vi "Login-Panel.vi"() -> ()   [LabVIEW 2021]
uses:
  <vilib>/lvdsc/security/NI Security Programmatic Login (Name).vi
  Global-Var-Simulator.vi
  <vilib>/lvdsc/NI_DSC.lvlib
panel:
  in  "goto_control_panel_btn":bool
  in  "logout_button":bool
  out "active_user_L":string
  in  "goto_service_panel_btn":bool
  in  "service_login_btn":bool
  in  "goto_wash_panel_btn":bool
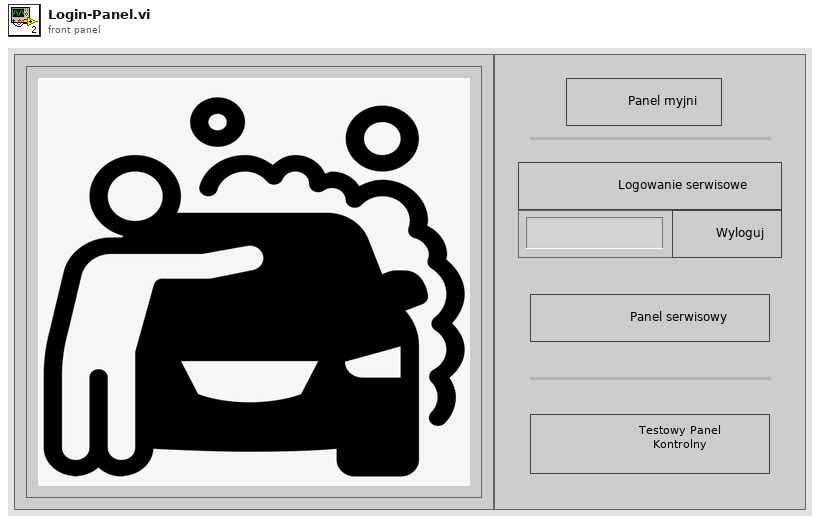
[diagram p1: front panel]
types:
  T1 = enum32{"Invalid", "Standard", "Closed", "Hidden", "Minimized", "Maximized"}
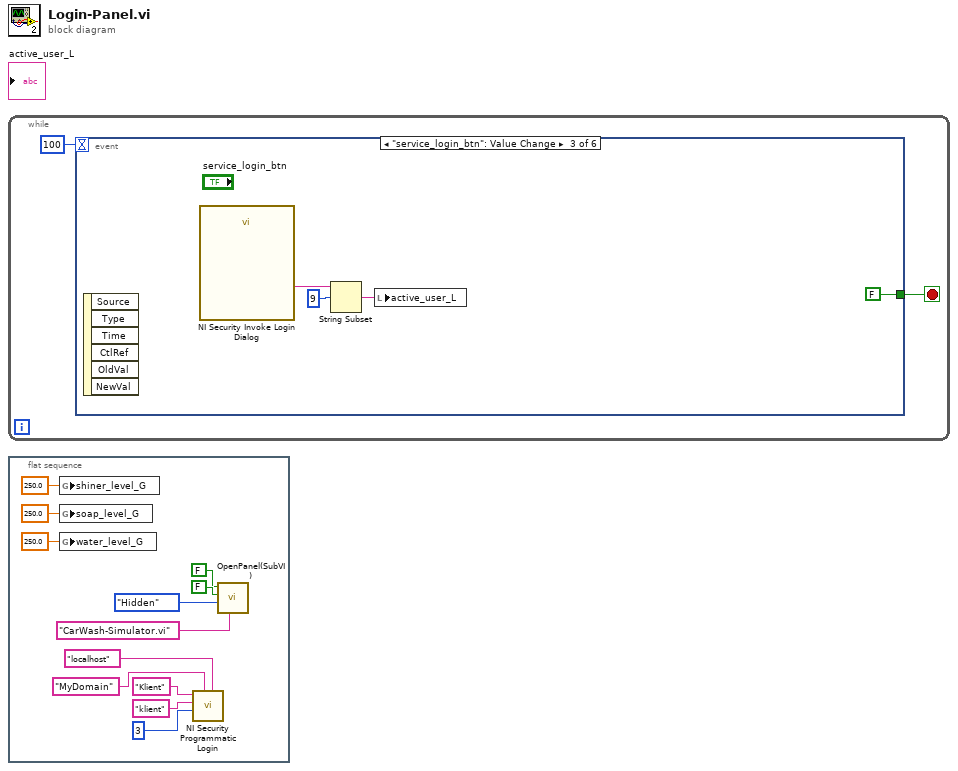
[diagram p0: block diagram]
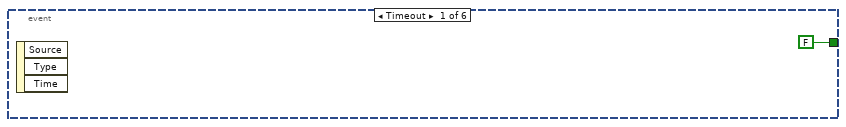
[diagram p2: hidden frame]
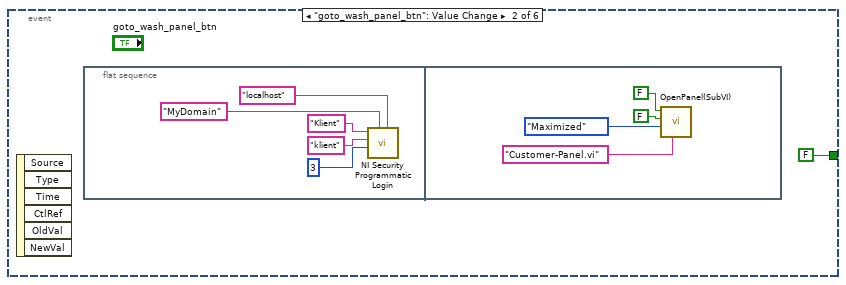
[diagram p3: hidden frame]
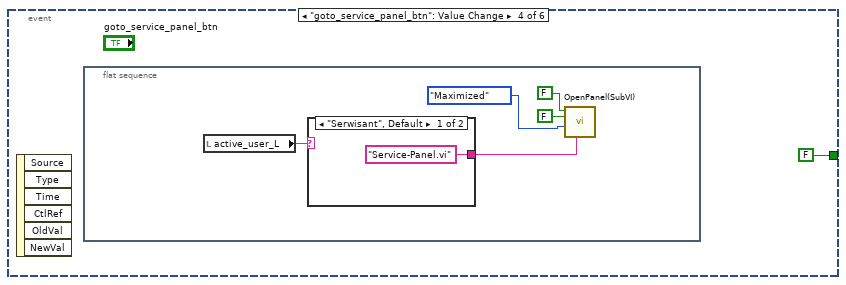
[diagram p4: hidden frame]
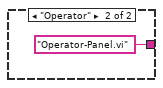
[diagram p5: hidden frame]
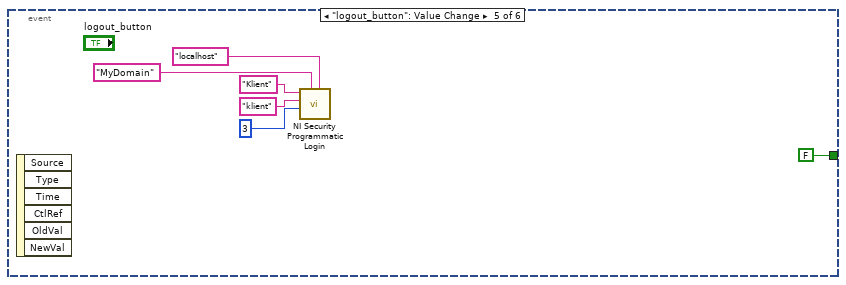
[diagram p6: hidden frame]
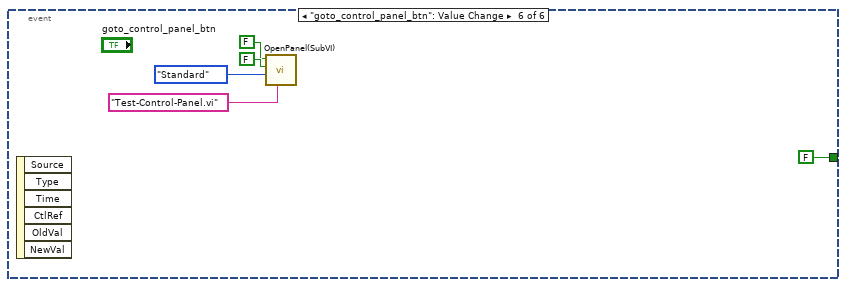
[diagram p7: hidden frame]
diagram:
  n1 = while {
    stop <- w1 stop-if-true
    n2 = event shown="[2] \"service_login_btn\": Value Change" {
      selector: _ -> [_ _ _ _ _ _]
      dyn-events: _ -> [_ _ _ _ _ _]
      timeout: 100 -> [_ _ _ _ _ _]
      tunnel: [FALSE FALSE FALSE FALSE FALSE FALSE] -> w1
      event Timeout {
        n3 = event-data() -> ()  [unwired: 1 in, 3 out]
      }
      event "goto_wash_panel_btn": Value Change {
        n4 = event-data() -> ()  [unwired: 1 in, 6 out]
        n5 = flat-sequence {
          frame #0 {
            n6 = call-poly <vilib>:"NI Security Programmatic Login.vi"("domain machine"="localhost", "domain name"="MyDomain", "timeout (30s)"=u32 3, "password"="klient", "user name"="Klient") -> ()  [unwired: 4 in, 3 out]
          }
          frame #1 {
            n7 = call "OpenPanel(SubVI).vi"("String"="Customer-Panel.vi", "State"=T1."Maximized", "Wait Until Done"=FALSE, "Auto Dispose Reference"=FALSE) -> ()  [unwired: 8 in]
          }
        }
      }
      event "service_login_btn": Value Change {
        n8 = event-data() -> ()  [unwired: 1 in, 6 out]
        n9 = call <vilib>:"NI Security Invoke Login Dialog.vi"() -> ("interactive user name"=w16:string)  [unwired: 8 in, 3 out]
        n10 = String Subset(string=w16, offset (0)=9) -> (substring=w15:string)  [unwired: 1 in]
        n11 = local write "active_user_L"(w15) -> ()
      }
      event "goto_service_panel_btn": Value Change {
        n12 = event-data() -> ()  [unwired: 1 in, 6 out]
        n13 = flat-sequence {
          frame #0 {
            n14 = local read "active_user_L"() -> (w22:string)
            n15 = case shown="\"Serwisant\", Default" w22 {
              tunnel: ["Service-Panel.vi" "Operator-Panel.vi"] -> w23
              frame "Serwisant", Default {
              }
              frame "Operator" {
              }
            }
            n16 = call "OpenPanel(SubVI).vi"("String"=w23, "State"=T1."Maximized", "Wait Until Done"=FALSE, "Auto Dispose Reference"=FALSE) -> ()  [unwired: 8 in]
          }
        }
      }
      event "logout_button": Value Change {
        n17 = event-data() -> ()  [unwired: 1 in, 6 out]
        n18 = call-poly <vilib>:"NI Security Programmatic Login.vi"("domain machine"="localhost", "domain name"="MyDomain", "timeout (30s)"=u32 3, "password"="klient", "user name"="Klient") -> ()  [unwired: 4 in, 3 out]
      }
      event "goto_control_panel_btn": Value Change {
        n19 = event-data() -> ()  [unwired: 1 in, 6 out]
        n20 = call "OpenPanel(SubVI).vi"("String"="Test-Control-Panel.vi", "State"=T1."Standard", "Wait Until Done"=FALSE, "Auto Dispose Reference"=FALSE) -> ()  [unwired: 8 in]
      }
    }
  }
  n21 = flat-sequence {
    frame #0 {
      n22 = global write "Global-Var-Simulator.vi" "shiner_level_G"(250.0 ("shiner_level_G")) -> ()
      n23 = global write "Global-Var-Simulator.vi" "soap_level_G"(250.0 ("soap_level_G")) -> ()
      n24 = global write "Global-Var-Simulator.vi" "water_level_G"(250.0 ("water_level_G")) -> ()
      n25 = call-poly <vilib>:"NI Security Programmatic Login.vi"("domain machine"="localhost", "domain name"="MyDomain", "timeout (30s)"=u32 3, "password"="klient", "user name"="Klient") -> ()  [unwired: 4 in, 3 out]
      n26 = call "OpenPanel(SubVI).vi"("String"="CarWash-Simulator.vi", "State"=T1."Hidden", "Wait Until Done"=FALSE, "Auto Dispose Reference"=FALSE) -> ()  [unwired: 8 in]
    }
  }
